vi "Move To Start Position Enabled.vi"(8 "error in (no error)":errorcluster {"code" format="%.0x"}, 9 "Enabled (True)":bool=TRUE, 10 "Device Number (1)":i32=1, 11 "VISA Resource Name":refnum<visa-resource-name>) -> (0 "error out":errorcluster {"code" format="%.0x"}, 3 "VISA Resource Name Out":refnum<visa-resource-name>)   [LabVIEW 2020, in "Olympus IX BX Series.lvlib"]
doc: "Sets / cancels returning operation to the start position after initializing the origin."
uses:
  Olympus IX BX Series.lvlib
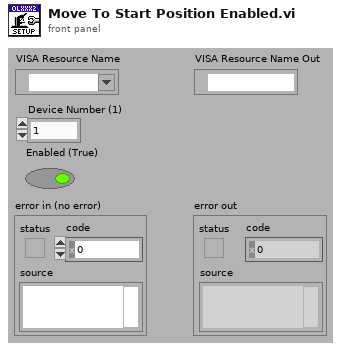
[diagram p1: front panel]
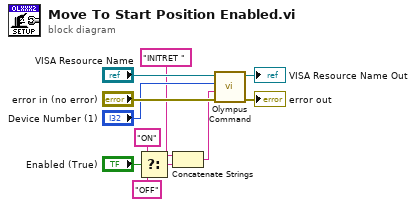
[diagram p0: block diagram]
diagram:
  n1 = Select(t="ON", s="Enabled (True)", f="OFF") -> (s? t:f=w3:string)
  n2 = Concatenate Strings("INITRET " ("format string"), w3) -> (w1:string)
  n3 = call "Olympus Command.vi"("error in (no error)"="error in (no error)", "Command string"=w1, "Device Number (1)"="Device Number (1)", "VISA Resource Name"="VISA Resource Name") -> ("error out"=→"error out":errorcluster, "VISA Resource Name Out"=→"VISA Resource Name Out":refnum<visa-resource-name>)  [unwired: 5 in, 1 out]
